vi "bead-centroid-darkfield.vi"(7 "Image Src":T1, 8 "error in (no error)":errorcluster, 9 "Image bw":T1, 10 "Image threshold":T1, 11 "Threshold Value":cluster{i32, i32}(slide)={0, 76} scale=0.0..255.0) -> (0 "error out":errorcluster, 1 "Image bw Out":T1, 2 "Image threshold Out":T1, 3 "Centroid":cluster{"X Centroid":sgl, "Y Centroid":sgl} {"Y Centroid" format="%.2f"; "X Centroid" format="%.2f"})   [LabVIEW 2013]
uses:
  <vilib>/vision/Image Controls.llb/IMAQ Image.ctl
  <vilib>/vision/NI_Vision_Development_Module.lvlib
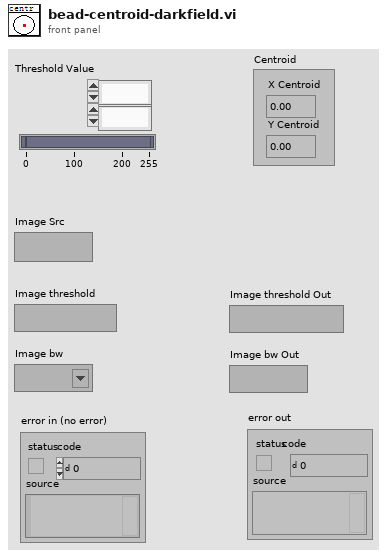
[diagram p1: front panel]
types:
  T1 = typedef "IMAQ Image.ctl" = refnum<image>
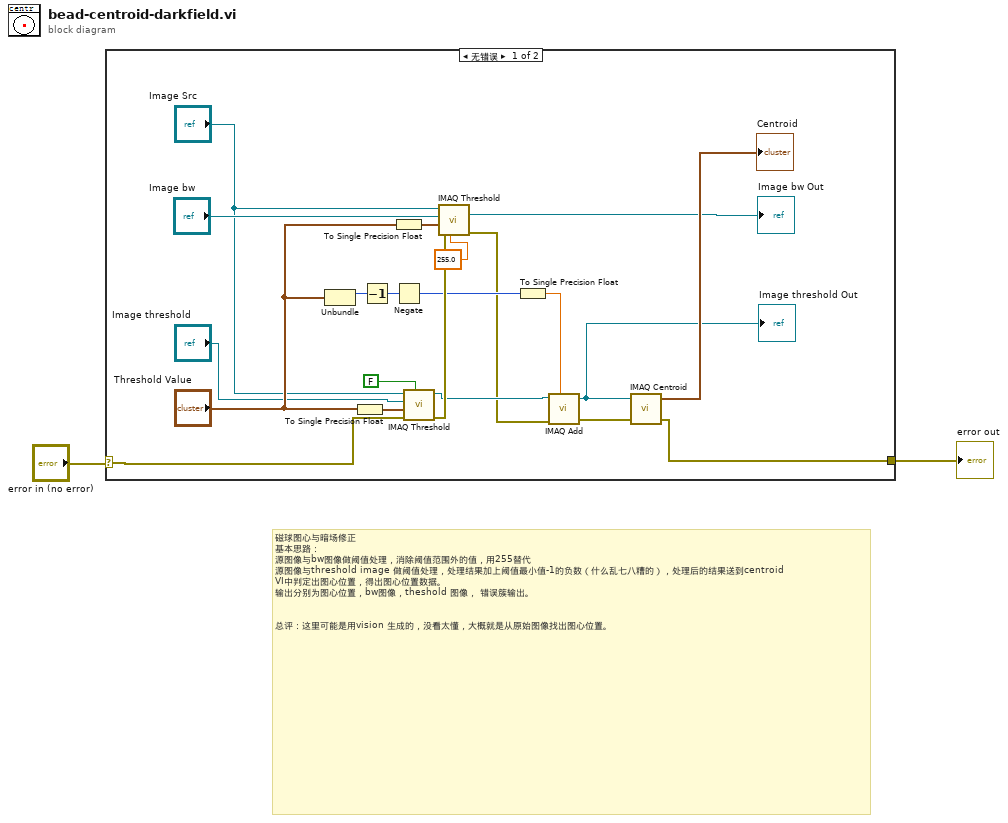
[diagram p0: block diagram]
diagram:
  # "磁球图心与暗场修正\n基本思路：\n源图像与bw图像做阈值处理，消除阈值范围外的值，用255替代\n源图像与threshold image 做阈值处理，处理结果加上阈值最小值-1的负数（什么乱七八糟的），处理后的结果送到centroid VI中判定出图心位置，得出图心位置数据。\n输出分别为图心位置，bw图像，theshold 图像， 错误簇输出。\n\n\n总评：这里可能是用vision 生成的，没看太懂，大概就是从原始图像找出图心位置。"
  n1 = case shown="无错误" "error in (no error)" {
    selector: "error in (no error)" -> [w6 w24]
    tunnel: [w8 w24] -> w2
    frame No Error {
      n2 = Unbundle("Threshold Value") -> (w14:i32)  [unwired: 1 out]
      n3 = To Single Precision Float(number="Threshold Value") -> (single precision float=w5:cluster{sgl, sgl})
      n4 = Decrement(x=w14) -> (x-1=w13:i32)
      n5 = To Single Precision Float(number="Threshold Value") -> (single precision float=w4:cluster{sgl, sgl})
      n6 = Negate(x=w13) -> (-x=w16:i32)
      n7 = call "IMAQ Threshold"("Keep/Replace Value (Replace)"=FALSE, "error in (no error)"=w6, "Range"=w5, "Image Dst"="Image threshold", "Image Src"="Image Src") -> ("error out"=w20:errorcluster, "Image Dst Out"=w17:T1)  [unwired: 5 in]
      n8 = call "IMAQ Threshold"("Replace Value"=sgl 255.0, "error in (no error)"=w20, "Range"=w4, "Image Dst"="Image bw", "Image Src"="Image Src") -> ("error out"=w15:errorcluster, "Image Dst Out"=→"Image bw Out":T1)  [unwired: 5 in]
      n9 = To Single Precision Float(number=w16) -> (single precision float=w3:sgl)
      n10 = call "IMAQ Add"("Image Src A"=w17, "Constant"=w3, "error in (no error)"=w15) -> ("Image Dst Out"=w7:T1, "error out"=w10:errorcluster)  [unwired: 2 in, 2 out]
      "Image threshold Out" <- w7
      n11 = call "IMAQ Centroid"("error in (no error)"=w10, "Image"=w7) -> ("error out"=w8:errorcluster, "Centroid"=→"Centroid":cluster{"X Centroid":sgl, "Y Centroid":sgl})  [unwired: 1 in, 1 out]
    }
    frame Error {
    }
  }
  "error out" <- w2
